vi "FIB image draw milling.vi"(0 "Milling Z Voltage":dbl, 3 "Milling para":T1={"X resolution"=4096, "Z resolution"=125001, "X offset (um)"=0.0, "Z offset (um)"=0.0, "X center (um)"=0.0, "Z center (um)"=0.0, "X size (um)"=250.0, "Z size (um)"=250.0, "UL-Ang"=90.0, "UR-Ang"=90.0, "Line milling time (s)"=5.0, "Z-step (nm)"=2.0, "Lines auto pause"=1, "Auto pause"=FALSE, "Mill from Bottom"=FALSE, "FIB FOV (um)"=500.0, "Auto Profile"=FALSE, "Mill start from Last"=FALSE, "FIB PID on"=FALSE, "FIB PID reset"=TRUE, "FIB PID measured"=0, "FIB PID target"=0.0, "FIB PID target slope"=0.0, "FIB PID P"=0.001, "FIB PID I"=0.01, "FIB PID D"=0.0, "Emission (uA)"=1.36, "Suppressor (V)"=50.0, "Auto reheat"=FALSE} caption="Milling Parameters" {"Suppressor (V)" step=0.1 format="%.1g"; "Emission (uA)" step=0.1 format="%.2g"; "FIB PID measured" items=["Spec.", "B.D. 1", "B.D. 2", "Mill", "Spec. +"]; "FIB PID target slope" min=-1 max=1 step=0.1; "UR-Ang" format="%.2f"; "UL-Ang" format="%.2f"; "Z offset (um)" step=0.02 format="%.3g"; "X offset (um)" step=1 format="%.3g"; "FIB FOV (um)" format="%.3g"; "Line milling time (s)" format="%.1f"; "Z center (um)" format="%#.3g"; "X center (um)" format="%#.3g"}, 4 "Z offset pre (um)":dbl, 8 "FIB Options":T3={"Scan mode"=0, "Flip x"=TRUE, "Flip z"=TRUE, "Det"=0} {"Scan mode" items=["Raster", "Serpentine"]; "Det" items=["Detector A", "Detector B"]}, 9 "FIB Scan Parameters":T2={"X resolution"=512, "Z resolution"=512, "X center"=0.0, "Z center"=0.0, "X size (V)"=10.0, "Z size (V)"=10.0, "Frame line rampdown ratio"=-0.1, "Scan rate (Hz)"=2000000, "Oversampling"=2} {"Z size (V)" min=0.0 max=20.0; "X size (V)" min=0.0 max=20.0; "Frame line rampdown ratio" min=-1.0 max=1.0 step=0.05 format="%.2g"; "Scan rate (Hz)" max=4000000 format="%#.6p"; "Z resolution" max=2048; "X resolution" max=2048}, 10 "Origin":bool, 11 "Image reference":refnum<vi>) -> (1 "X size factor":dbl, 2 "Trapezoidal":cluster{"X":i16, "Y":i16}[](array[cluster]))   [LabVIEW 2018]
panel:
  # "Direction"
  # "Start\nfrom"
  # "<"
  # "Flip"
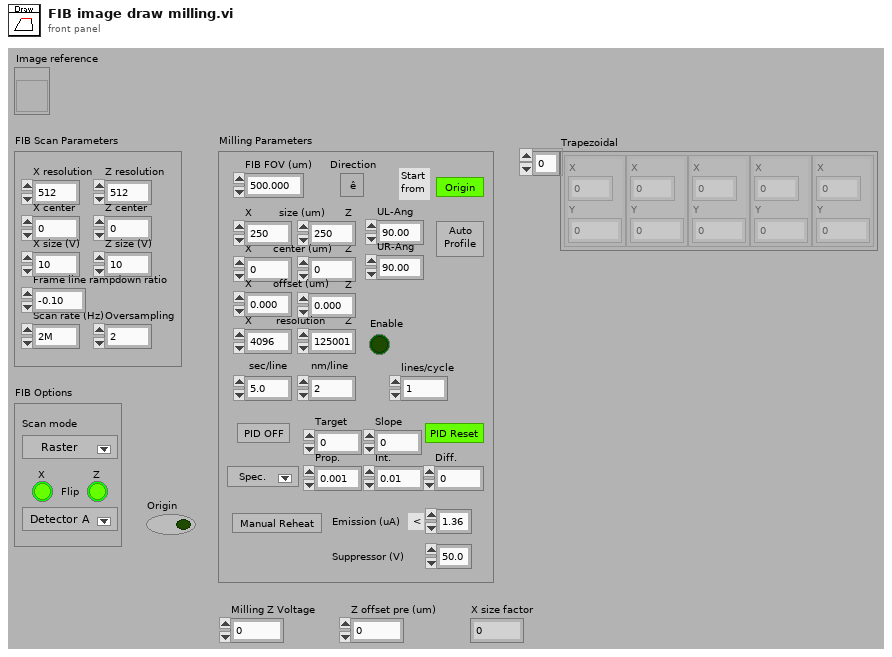
[diagram p1: front panel]
types:
  T1 = cluster{"X resolution":u32, "Z resolution":u32, "X offset (um)":sgl, "Z offset (um)":sgl, "X center (um)":sgl, "Z center (um)":sgl, "X size (um)":sgl, "Z size (um)":sgl, "UL-Ang":sgl, "UR-Ang":sgl, "Line milling time (s)":sgl, "Z-step (nm)":dbl, "Lines auto pause":u16, "Auto pause":bool, "Mill from Bottom":bool, "FIB FOV (um)":sgl, "Auto Profile":bool, "Mill start from Last":bool, "FIB PID on":bool, "FIB PID reset":bool, "FIB PID measured":u8, "FIB PID target":sgl, "FIB PID target slope":sgl, "FIB PID P":sgl, "FIB PID I":sgl, "FIB PID D":sgl, "Emission (uA)":dbl, "Suppressor (V)":sgl, "Auto reheat":bool}
  T2 = cluster{"X resolution":u32, "Z resolution":u32, "X center":dbl, "Z center":dbl, "X size (V)":dbl, "Z size (V)":dbl, "Frame line rampdown ratio":dbl, "Scan rate (Hz)":u32, "Oversampling":u16}
  T3 = cluster{"Scan mode":u16, "Flip x":bool, "Flip z":bool, "Det":u16}
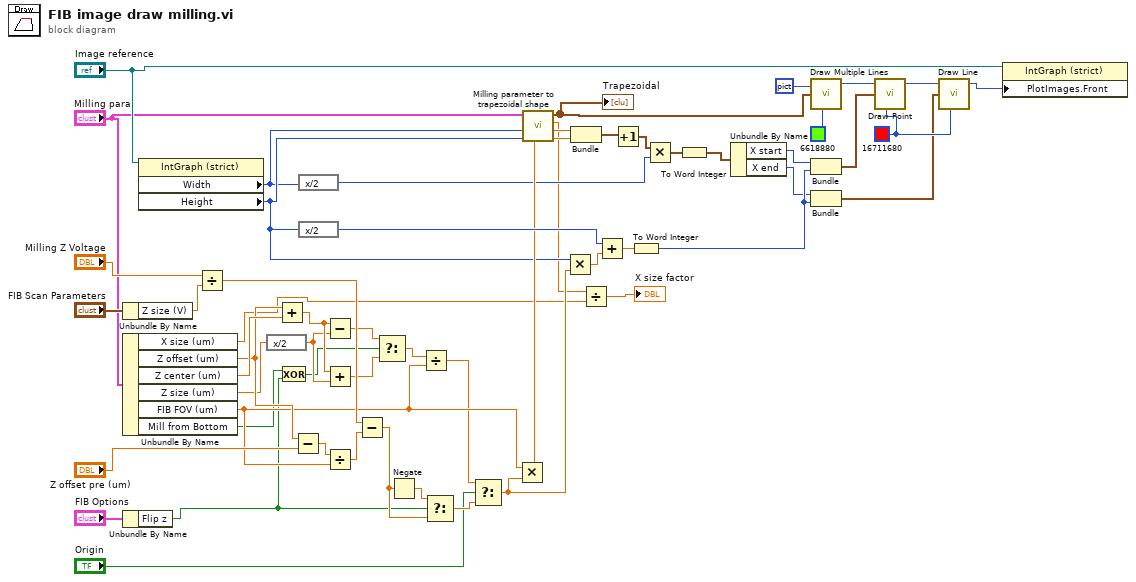
[diagram p0: block diagram]
diagram:
  w48 = u32 16711680 ("color(black)")
  n1 = Unbundle By Name("FIB Scan Parameters") -> ("Z size (V)"=w30:dbl)
  n2 = Unbundle By Name("Milling para") -> ("X size (um)"=w3:sgl, "Z offset (um)"=w19:sgl, "Z center (um)"=w20:sgl, "Z size (um)"=w18:sgl, "FIB FOV (um)"=w11:sgl, "Mill from Bottom"=w7:bool)
  n3 = Unbundle By Name("FIB Options") -> ("Flip z"=w6:bool)
  n4 = property on="Property Node" class="IntGraph (strict)"(reference="Image reference") -> ("Width"=w37:u32, "Height"=w41:u32)  [unwired: 1 in, 2 out]
  n5 = Divide(x="Milling Z Voltage", y=w30) -> (x/y=w24:dbl)
  n6 = expression code="x/2"(w18) -> (w16:sgl)
  n7 = Add(x=w19, y=w20) -> (x+y=w17:sgl)
  n8 = Exclusive Or(1:w6, 2:w7) -> (0:w15:bool)
  n9 = Subtract(x=w19, y="Z offset pre (um)") -> (x-y=w25:dbl)
  n10 = expression code="x/2"(w37) -> (w35:u32)
  n11 = expression code="x/2"(w41) -> (w51:u32)
  n12 = Subtract(x=w17, y=w16) -> (x-y=w13:sgl)
  n13 = Add(x=w17, y=w16) -> (x+y=w14:sgl)
  n14 = Divide(x=w25, y=w11) -> (x/y=w22:dbl)
  n15 = Subtract(x=w24, y=w22) -> (x-y=w23:dbl)
  n16 = Select(t=w13, s=w15, f=w14) -> (s? t:f=w12:sgl)
  n17 = Negate(x=w23) -> (-x=w44:dbl)
  n18 = Divide(x=w12, y=w11) -> (x/y=w8:sgl)
  n19 = Select(t=w44, s=w6, f=w23) -> (s? t:f=w9:dbl)
  n20 = Select(t=w8, s="Origin", f=w9) -> (s? t:f=w10:dbl)
  n21 = Multiply(x=w11, y=w10) -> (x*y=w43:dbl)
  n22 = call "Milling parameter to trapezoidal shape.vi"("Y location (um)"=w43, "Image height"=w41, "Image width"=w37, "Milling para"="Milling para") -> ("X end"=w39:dbl, "X start"=w40:dbl, "X size (um) @ Y"=w4:dbl, "Trapezoidal"=w42:cluster{"X":i16, "Y":i16}[])  [unwired: 3 in, 1 out]
  "Trapezoidal" <- w42
  n23 = Multiply(x=w41, y=w10) -> (x*y=w52:dbl)
  n24 = Bundle("X start"=w40, "X end"=w39) -> (w38:cluster{"X start":dbl, "X end":dbl})  [unwired: 1 in]
  n25 = Divide(x=w4, y=w3) -> (x/y=→"X size factor":dbl)
  n26 = Add(x=w51, y=w52) -> (x+y=w50:dbl)
  n27 = Increment(x=w38) -> (x+1=w36:cluster{"X start":dbl, "X end":dbl})
  n28 = To Word Integer(number=w50) -> (16bit integer=w47:i16)
  n29 = Multiply(x=w36, y=w35) -> (x*y=w34:cluster{"X start":dbl, "X end":dbl})
  n30 = To Word Integer(number=w34) -> (16bit integer=w33:cluster{"X start":i16, "X end":i16})
  n31 = Unbundle By Name(w33) -> ("X start"=w32:i16, "X end"=w31:i16)
  n32 = call <vilib>:"Draw Multiple Lines.vi"("picture"=picture data[5B], "line endpoints"=w42, "color(black)"=u32 6618880) -> ("new picture"=w54:picture)  [unwired: 6 in]
  n33 = Bundle("X start"=w32, w47) -> (w49:cluster{"X start":i16, i16})  [unwired: 1 in]
  n34 = Bundle("X end"=w31, w47) -> (w46:cluster{"X end":i16, i16})  [unwired: 1 in]
  n35 = call <vilib>:"Draw Point.vi"("picture"=w54, "point(x,y)"=w49, "color(black)"=w48) -> ("new picture"=w53:picture)  [unwired: 6 in]
  n36 = call <vilib>:"Draw Line.vi"("picture"=w53, "end point"=w46, "color(black)"=w48) -> ("new picture"=w45:picture)  [unwired: 6 in]
  n37 = property on="Property Node" class="IntGraph (strict)"(reference="Image reference", "PlotImages.Front"=w45) -> ()  [unwired: 1 in, 2 out]
